vi "Init.vi"(0 "Experiment3D in":refnum<class "Experiment3D.lvclass">, 5 "Measurement3D.lvclass":refnum<class "Measurement3D.lvclass">, 7 "Data3D.lvclass":refnum<class "Data3D.lvclass">, 9 "Path":path, 11 "error in (no error)":errorcluster) -> (4 "Experiment3D out":refnum<class "Experiment3D.lvclass">, 15 "error out":errorcluster)   [LabVIEW 2014, in "Experiment3D.lvclass"]
uses:
  Experiment3D.lvclass
  Measurement/Measurement3D/Measurement3D.lvclass
  Instrument/Instrument/Instrument.lvclass
  Data/Data3D/Data3D.lvclass
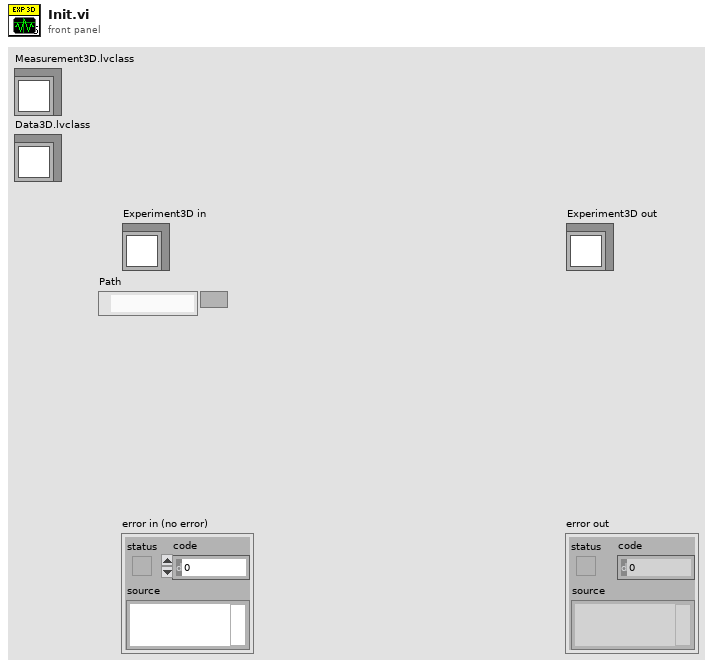
[diagram p1: front panel]
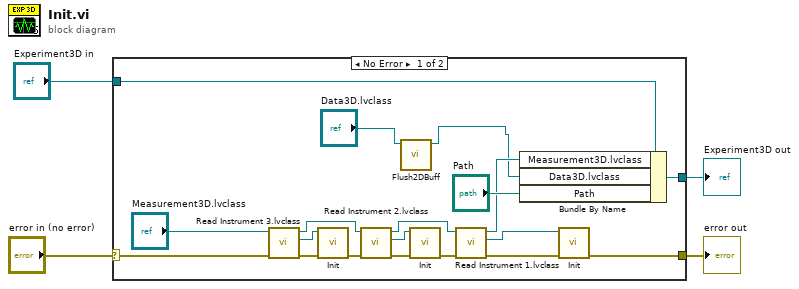
[diagram p0: block diagram]
diagram:
  n1 = case shown="No Error" "error in (no error)" {
    selector: "error in (no error)" -> [w9 w25]
    tunnel: [w7 w25] -> w3
    tunnel: [w10 w24] -> w1
    tunnel: "Experiment3D in" -> [w11 w24]
    frame No Error {
      n2 = call "Read Instrument 3.lvclass.vi"("error in (no error)"=w9, "Measurement3D in"="Measurement3D.lvclass") -> ("error out"=w17:errorcluster, "Instrument.lvclass"=w18:refnum<class "Instrument.lvclass">, "Measurement3D out"=w21:refnum<class "Measurement3D.lvclass">)  [unwired: 7 in]
      n3 = call-dynamic "Init.vi"("error in (no error)"=w17, "Instrument in"=w18) -> ("error out"=w16:errorcluster)  [unwired: 8 in, 1 out]
      n4 = call "Read Instrument 2.lvclass.vi"("error in (no error)"=w16, "Measurement3D in"=w21) -> ("error out"=w14:errorcluster, "Instrument.lvclass"=w15:refnum<class "Instrument.lvclass">, "Measurement3D out"=w20:refnum<class "Measurement3D.lvclass">)  [unwired: 7 in]
      n5 = call "Flush2DBuff.vi"("Data3D in"="Data3D.lvclass") -> ("Data3D out"=w5:refnum<class "Data3D.lvclass">)  [unwired: 9 in, 1 out]
      n6 = call-dynamic "Init.vi"("error in (no error)"=w14, "Instrument in"=w15) -> ("error out"=w13:errorcluster)  [unwired: 8 in, 1 out]
      n7 = call "Read Instrument 1.lvclass.vi"("error in (no error)"=w13, "Measurement3D in"=w20) -> ("error out"=w8:errorcluster, "Instrument.lvclass"=w12:refnum<class "Instrument.lvclass">, "Measurement3D out"=w19:refnum<class "Measurement3D.lvclass">)  [unwired: 7 in]
      n8 = Bundle By Name(cluster=w11, "Measurement3D.lvclass"=w19, "Data3D.lvclass"=w5, "Path"="Path") -> (w10:refnum<class "Experiment3D.lvclass">)
      n9 = call-dynamic "Init.vi"("error in (no error)"=w8, "Instrument in"=w12) -> ("error out"=w7:errorcluster)  [unwired: 8 in, 1 out]
    }
    frame Error {
    }
  }
  "error out" <- w3
  "Experiment3D out" <- w1
